vi "Analyze_VIs.vi"(7 "LabVIEW Web Service Request":refnum<class "Web Request.lvclass">, 11 "JSON":string) -> (3 "Result":string)   [LabVIEW 2014]
uses:
  <vilib>/wsapi/Web Request.lvclass
  <vilib>/wsapi/NI_WebServices.lvlib
  VI Analyzer/VI Analyzer.lvclass
panel:
  out "error out":errorcluster
  # "Use the Web Service Request input terminal to call the VIs on the Web Services palette. Do not remove it from the connector pane unless you don't need access to the palette."
  # "Each additional control wired to the connector pane will be available as an input in the URL. To include an indicator in terminal-mode output (the default setting), it must also be wired to the connector pane."
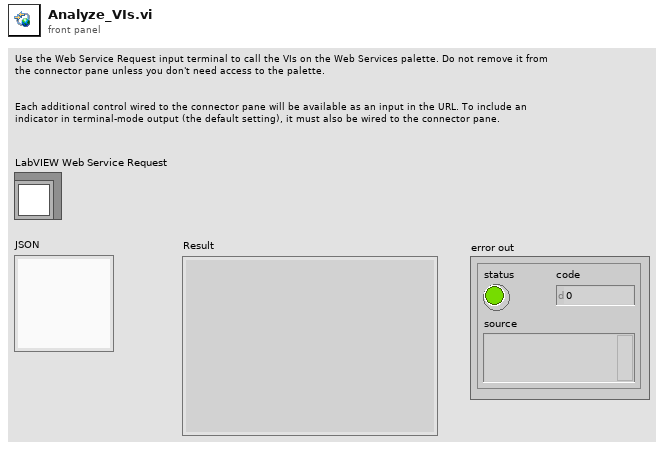
[diagram p1: front panel]
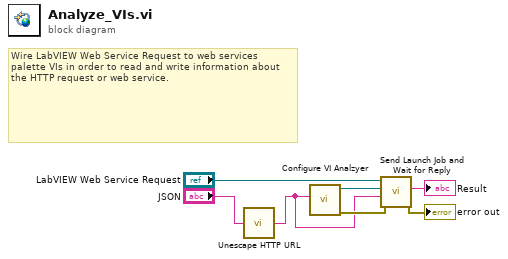
[diagram p0: block diagram]
diagram:
  # "Wire LabVIEW Web Service Request to web services palette VIs in order to read and write information about the HTTP request or web service."
  n1 = call <vilib>:"Unescape HTTP URL.vi"("escaped string in"="JSON") -> ("unescaped string out"=w1:string)
  n2 = call "Configure VI Analzyer.vi"("JSON String"=w1) -> ("error out"=w2:errorcluster, "VI Analyzer out"=w3:refnum<class "VI Analyzer.lvclass">)  [unwired: 9 in]
  n3 = call "Send Launch Job and Wait for Reply.vi"("error in (no error)"=w2, "JSON"=w1, "Job"=w3, "Web Request in"="LabVIEW Web Service Request") -> ("error out"=→"error out":errorcluster, "Result String"=→"Result":string)  [unwired: 6 in]
